vi "发送MES数据H.vi"(8 "error in (no error)":errorcluster caption="错误输入（无错误）", 10 "Data(IN)":string caption="DATA(IN)", 11 "MES配置":T1) -> (2 "RESULT":cluster{"Result":bool, "Message":string}, 3 "x = y?":bool, 4 "body 2":string caption="体部", 6 "headers":string caption="头部")   [LabVIEW 2014]
uses:
  <vilib>/regexp/Match Regular Expression.xnode
  <vilib>/httpClient/LabVIEWHTTPClient.lvlib
  <vilib>/httpClient/POSTBuffer.vi
panel:
  out "error out":errorcluster caption="错误输出"
  out "source":string caption="源"
  out "结果字符串":string
  out "body 3":string caption="体部"
  out "headers 3":string caption="头部"
  out "body":string caption="体部"
  out "headers 2":string caption="头部"
  out "Result":bool
  out "Message":string
  # "HTTP/1.1 200 OK\nDate: Wed, 25 Apr 2018 07:47:41 GMT\nSet-Cookie: JSESSIONID=642E0F2914D20608D4BB2EEA52589943.jvm3; Path=/sm5200/; HttpOnly\nContent-Type: text/html;charset=UTF-8\nContent-Length: 2619\nConnection: close"
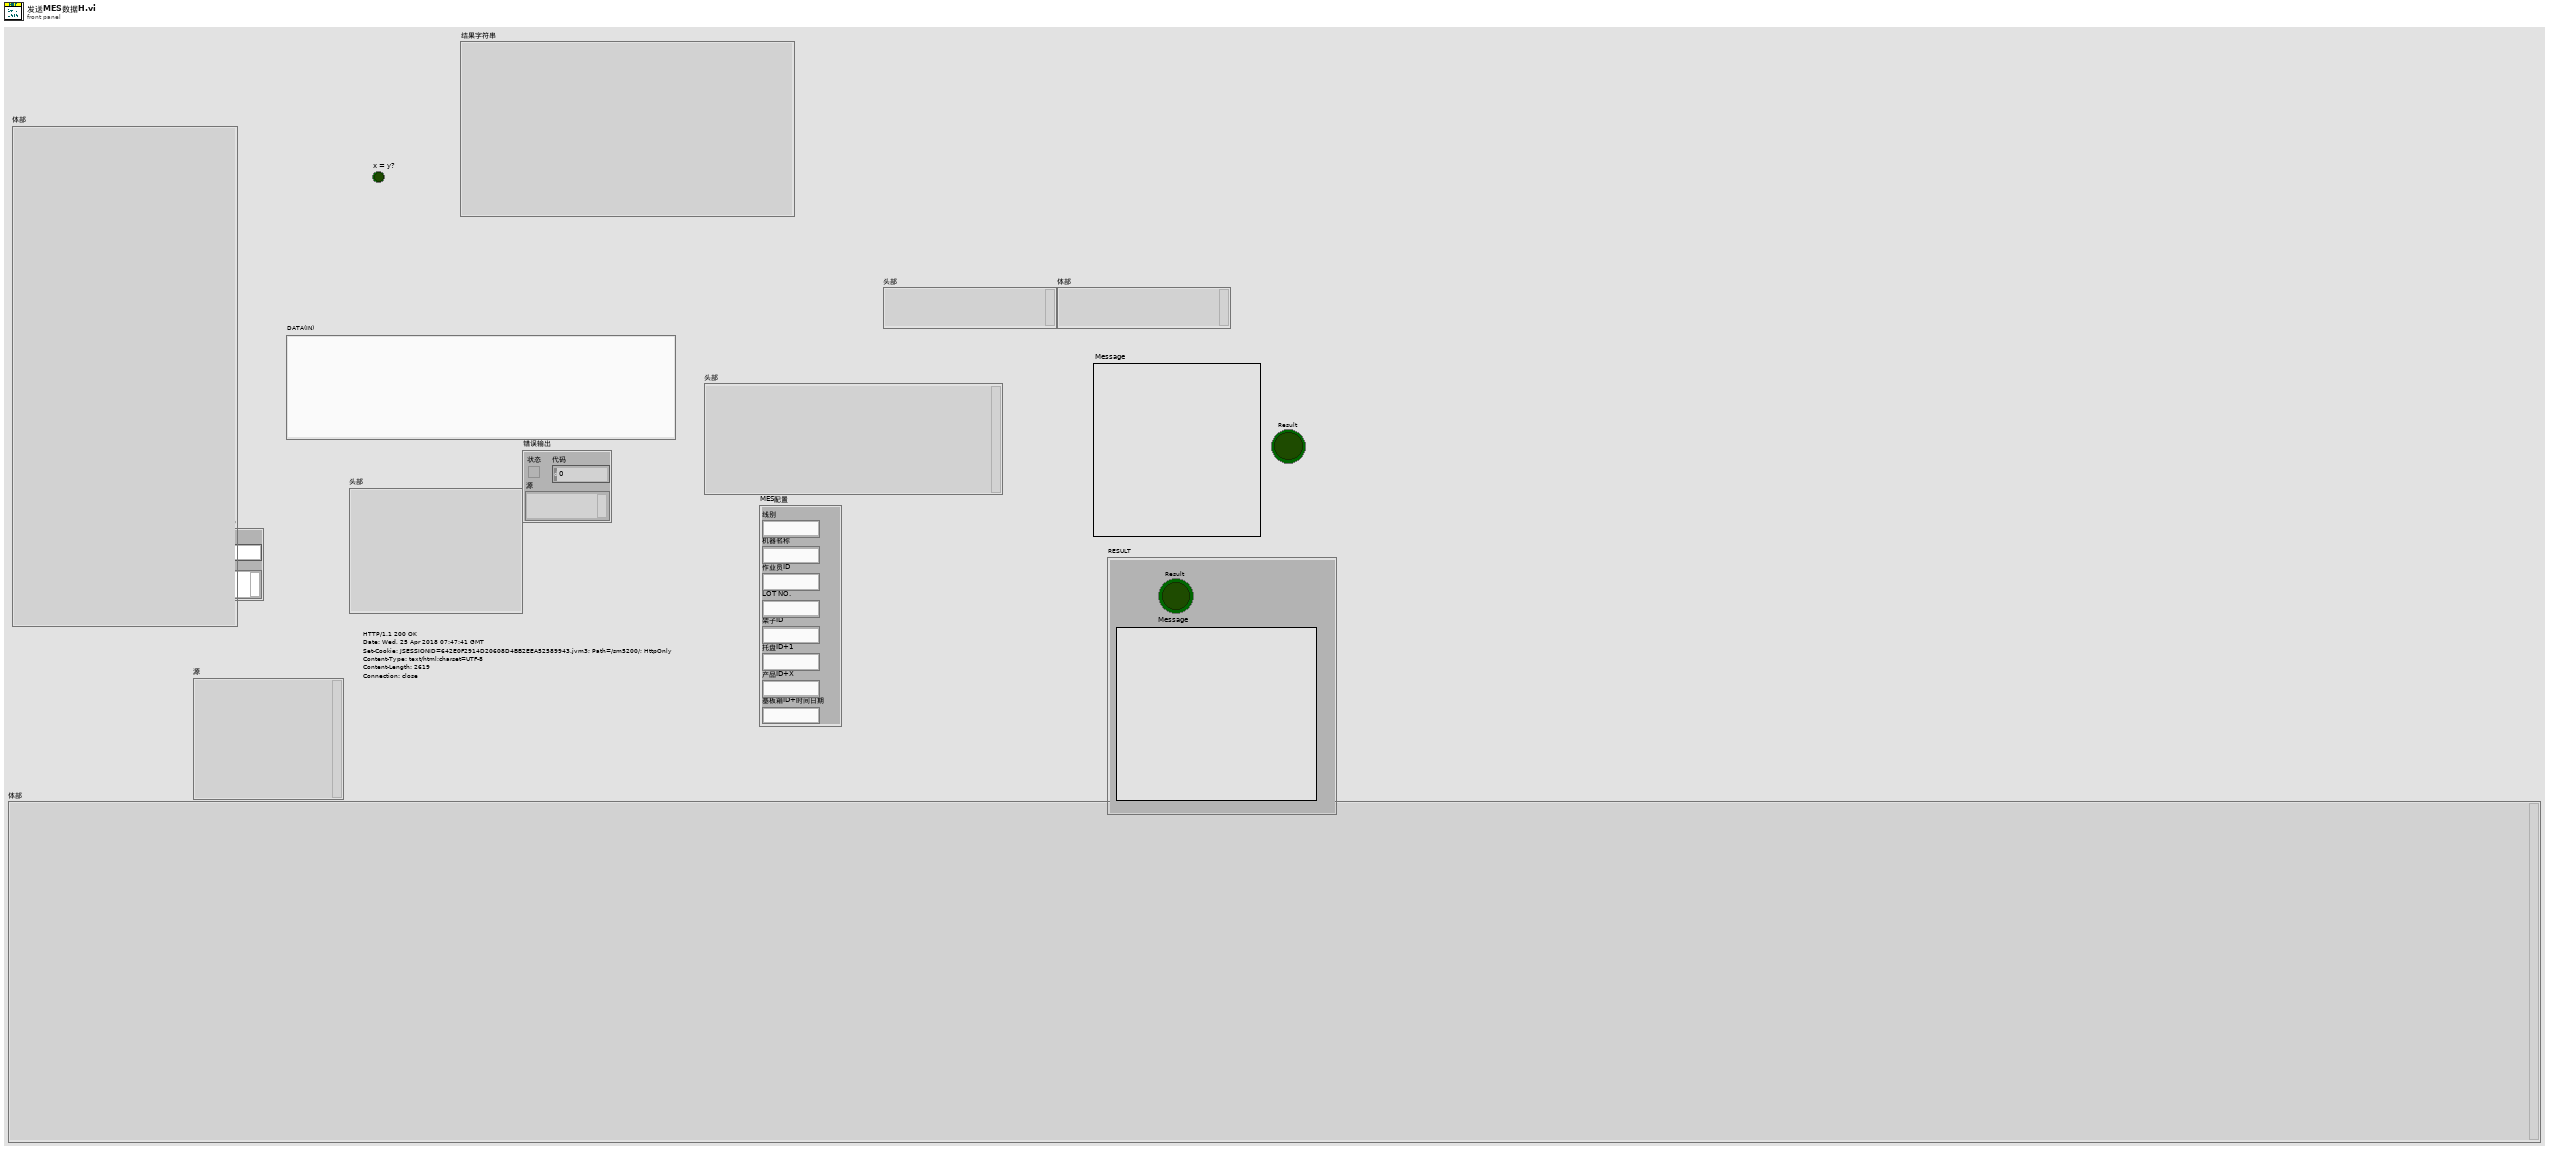
[diagram p1: front panel]
types:
  T1 = cluster{"线别":string, "机器名称":string, "作业员ID":string, "LOT NO.":string, "架子ID":string, "托盘ID+1":string, "产品ID+X":string, "基板箱ID+时间日期":string}
  T2 = typedef "LabVIEWHTTPClient.lvlib/ClientHandle.ctl" = refnum<k1>
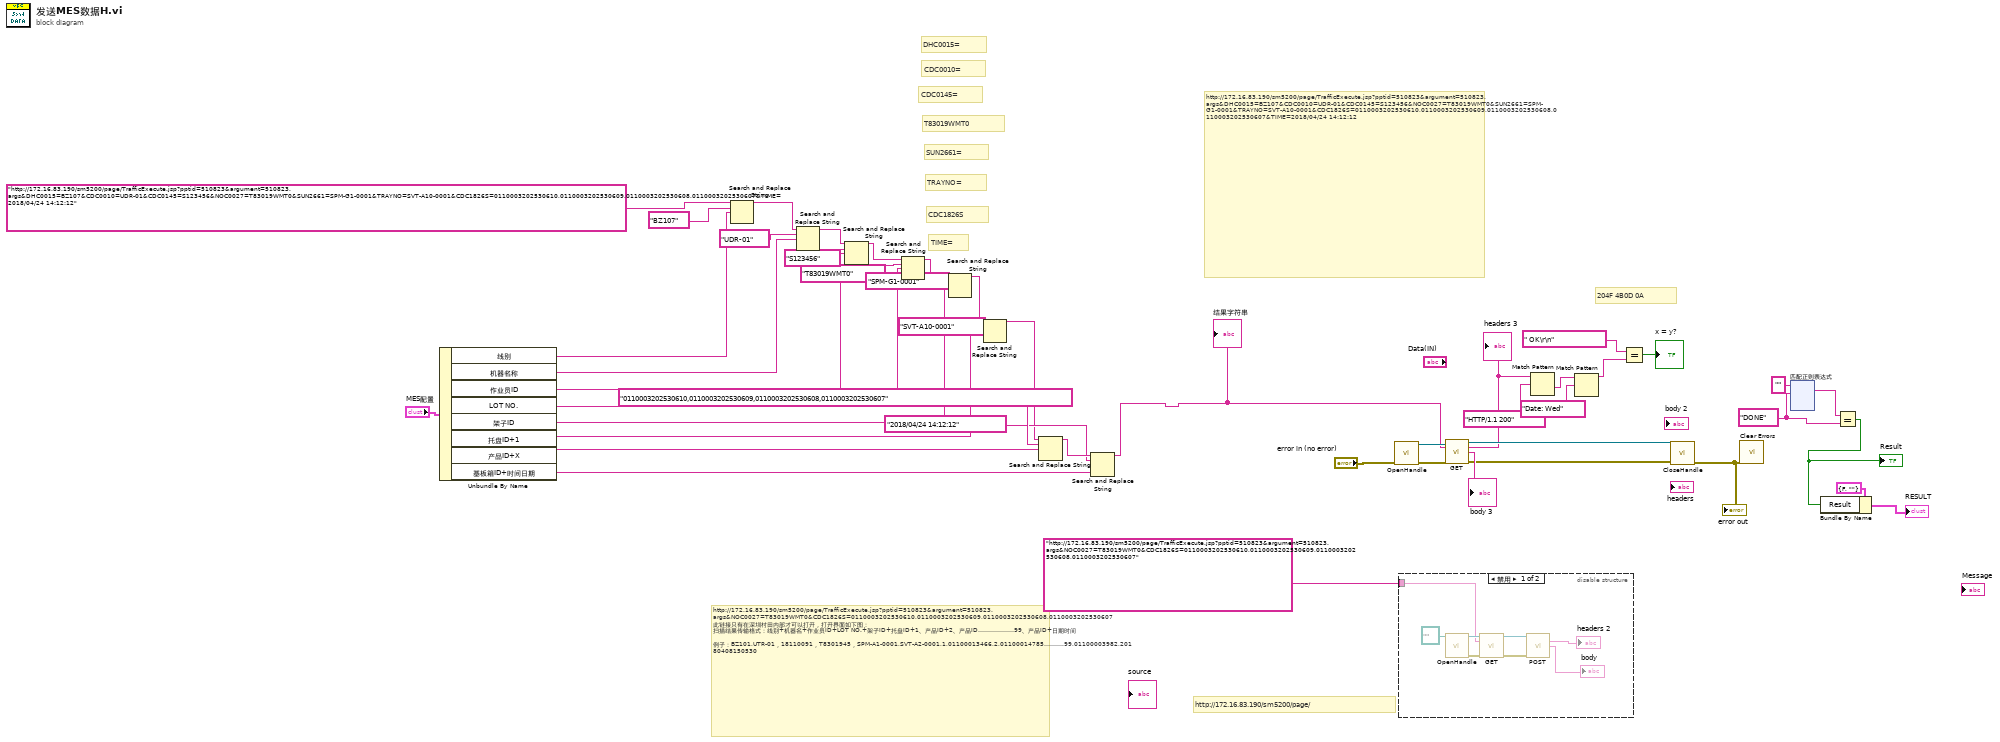
[diagram p0: block diagram]
diagram:
  w43 = "DONE"
  # "204F 4B0D 0A"
  # "TIME="
  # "CDC1826S"
  # "TRAYNO="
  # "SUN2661="
  # "T83019WMT0"
  # "CDC0145="
  # "CDC0010="
  # "DHC0015="
  # "http://172.16.83.190/sm5200/page/TrafficExecute.jsp?pptid=510823&argument=510823.args&DHC0015=BZ107&CDC0010=UDR-01&CDC0145=S123456&NOC0027=T83019WMT0&SUN2661=SPM-G1-0001&TRAYNO=SVT-A10-0001&CDC1826S=0110003202530610,0110003202530609,0110003202530608,0110003202530607&TIME=2018/04/24 14:12:12"
  # "http://172.16.83.190/sm5200/page/"
  # "http://172.16.83.190/sm5200/page/TrafficExecute.jsp?pptid=510823&argument=510823.args&NOC0027=T83019WMT0&CDC1826S=0110003202530610,0110003202530609,0110003202530608,0110003202530607\n此链接只有在深圳村田内部才可以打开，打开界面如下图：\n扫描结果传输格式：线别+机器名+作业员ID+LOT NO.+架子ID+托盘ID+1、产品ID+2、产品ID………………99、产品ID+日期时间\n                             例子：BZ101,UTR-01，18110091，T8301945，SPM-A1-0001,SVT-A2-0001,1,01100013466,2,01100014785……….99,01100003982,20180408150530"
  n1 = Unbundle By Name("MES配置") -> ("线别"=w34:string, "机器名称"=w31:string, "作业员ID"=w28:string, "LOT NO."=w25:string, "架子ID"=w22:string, "托盘ID+1"=w16:string, "产品ID+X"=w14:string, "基板箱ID+时间日期"=w13:string)
  n2 = Search and Replace String(input string="http://172.16.83.190/sm5200/page/TrafficExecute.jsp?pptid=510823&argument=510823.args&DHC0015=BZ107&CDC0010=UDR-01&CDC0145=S123456&NOC0027=T83019WMT0&SUN2661=SPM-G1-0001&TRAYNO=SVT-A10-0001&CDC1826S=0110003202530610,0110003202530609,0110003202530608,0110003202530607&TIME=2018/04/24 14:12:12" ("url"), search string="BZ107" ("替换字符串(\"\")"), replace string=w34) -> (result string=w33:string)  [unwired: 5 in, 3 out]
  n3 = Search and Replace String(input string=w33, search string="UDR-01" ("替换字符串(\"\")"), replace string=w31) -> (result string=w30:string)  [unwired: 5 in, 3 out]
  n4 = Search and Replace String(input string=w30, search string="S123456" ("搜索字符串"), replace string=w28) -> (result string=w27:string)  [unwired: 5 in, 3 out]
  n5 = Search and Replace String(input string=w27, search string="T83019WMT0" ("搜索字符串"), replace string=w25) -> (result string=w24:string)  [unwired: 5 in, 3 out]
  n6 = Search and Replace String(input string=w24, search string="SPM-G1-0001" ("搜索字符串"), replace string=w22) -> (result string=w18:string)  [unwired: 5 in, 3 out]
  n7 = Search and Replace String(input string=w18, search string="SVT-A10-0001" ("搜索字符串"), replace string=w16) -> (result string=w15:string)  [unwired: 5 in, 3 out]
  n8 = Search and Replace String(input string=w15, search string="0110003202530610,0110003202530609,0110003202530608,0110003202530607" ("搜索字符串"), replace string=w14) -> (result string=w20:string)  [unwired: 5 in, 3 out]
  n9 = Search and Replace String(input string=w20, search string="2018/04/24 14:12:12" ("搜索字符串"), replace string=w13) -> (result string=w8:string)  [unwired: 5 in, 3 out]
  "结果字符串" <- w8
  n10 = call <vilib>:"OpenHandle.vi"("error in (no error)"="error in (no error)") -> ("client handle out"=w40:T2, "error out"=w39:errorcluster)  [unwired: 13 in]
  n11 = disable-structure shown="禁用" {
    disable-tunnel: "http://172.16.83.190/sm5200/page/TrafficExecute.jsp?pptid=510823&argument=510823.args&NOC0027=T83019WMT0&CDC1826S=0110003202530610,0110003202530609,0110003202530608,0110003202530607" ("url") -> [w52 _]
    frame Disabled {
      n12 = call <vilib>:"OpenHandle.vi"("cookie file"=path "") -> ("client handle out"=w55:T2, "error out"=w54:errorcluster)  [unwired: 13 in]
      n13 = call <vilib>:"GET.vi"("client handle"=w55, "url"=w52, "error in (no error)"=w54) -> ("client handle out"=w51:T2, "error out"=w50:errorcluster)  [unwired: 9 in, 2 out]
      n14 = call-poly <vilib>:"POST.vi"("client handle"=w51, "error in (no error)"=w50) -> ("headers"=→"headers 2":string, "body"=→"body":string)  [unwired: 10 in, 2 out]
    }
    frame Enabled {
    }
  }
  n15 = call <vilib>:"GET.vi"("client handle"=w40, "url"=w8, "error in (no error)"=w39) -> ("client handle out"=w12:T2, "headers"=w7:string, "body"=→"body 3":string, "error out"=w11:errorcluster)  [unwired: 9 in]
  "headers 3" <- w7
  n16 = Match Pattern(string=w7, regular expression="HTTP/1.1 200" ("正则表达式")) -> (after substring=w5:string)  [unwired: 1 in, 3 out]
  n17 = Match Pattern(string=w5, regular expression="Date: Wed" ("正则表达式")) -> (before substring=w3:string)  [unwired: 1 in, 3 out]
  n18 = Equal?(x=" OK\r\n", y=w3) -> (x = y?=→"x = y?":bool)
  n19 = call <vilib>:"CloseHandle.vi"("client handle"=w12, "error in (no error)"=w11) -> ("error out"=w9:errorcluster)  [unwired: 13 in]
  "error out" <- w9
  n20 = call <vilib>:"Clear Errors.vi"("error in (no error)"=w9) -> ()  [unwired: 5 in, 2 out]
  n21 = xnode "匹配正则表达式"("输入字符串"="", "正则表达式"=w43) -> ("所有匹配"=w44:string)  [unwired: 4 in, 4 out]
  n22 = Equal?(x=w44, y=w43) -> (x = y?=w42:bool)
  "Result" <- w42
  n23 = Bundle By Name(cluster=cluster{"Result":bool, "Message":string} {"Result"=FALSE, "Message"=""} ("RESULT"), "Result"=w42) -> (→"RESULT":cluster{"Result":bool, "Message":string})
